vi "zmq_recv_multi.vi"(3 "error in":errorcluster, 5 "socket in":refnum<class "zmq_socket.lvclass">) -> (0 "error out":errorcluster, 1 "parts":string[](array[string]), 2 "socket out":refnum<class "zmq_socket.lvclass">)   [LabVIEW 2019, in "zeromq.lvlib" / "zmq_socket.lvclass"]
doc: "Receive a multi-component message from the socket. The incoming messages are returned as an array of strings, with one string for each message part.\n\nIf <b>no block?</b> is True, the function call will return immediately. Use zmq_check_timeout to see if it was simply a timeout or an error occurred.\n\nOtherwise this call will block until <b>all</b> parts of the message are received, an error is raised, or the socket is closed.\n\nNote there is no penalty using this function to receive single-part messages.\n\nDetailed API documentation: http://api.zeromq.org/3-2:zmq-recv"
uses:
  zmq_socket.lvclass
  zmq_socket.lvclass/zmq_socket.ctl
  <vilib>/Utility/error.llb/Error Cluster From Error Code.vi
  zeromq.lvlib
panel:
  # "ØMQ"
  # "labview"
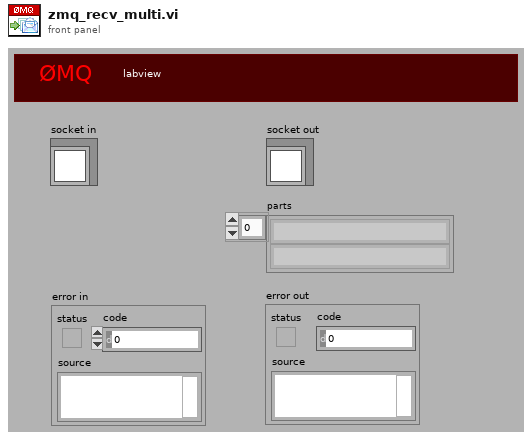
[diagram p1: front panel]
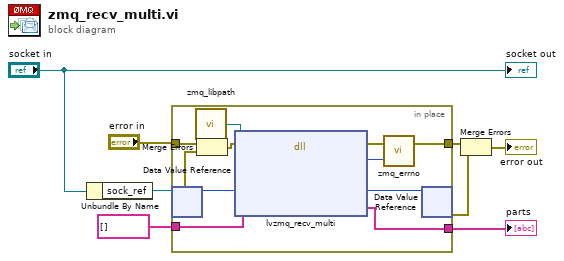
[diagram p0: block diagram]
diagram:
  n1 = Unbundle By Name("socket in") -> ("sock_ref"=w4:refnum<data-value>)
  n2 = in-place {
    in-place-border: "error in" -> [w17]
    in-place-border: [w16] -> w7
    in-place-border: string[] [] ("parts") -> [w15]
    in-place-border: [w12] -> w3
    n3 = in-place-dvr #1(w4) -> (w14:u64, w9:errorcluster)
    n4 = call "zmq_libpath.vi"() -> ("path"=w11:path)
    n5 = Merge Errors(w17, w9) -> (w10:errorcluster)
    n6 = dll-call lib="?" fn="lvzmq_recv_multi" ("zmq_labview.dll:lvzmq_socket")(path in=w11, error in=w10, "sock_obj"=w14, "data"=w15) -> (error out=w19:errorcluster, "return type"=w18:i32, "sock_obj"=w13:u64, "data"=w12:string[])  [unwired: 3 in, 1 out]
    n7 = call "zmq_errno.vi"("retval"=w18, "error in"=w19) -> ("error out"=w16:errorcluster)  [unwired: 1 out]
    n8 = in-place-dvr #1(w13) -> (w1:errorcluster)  [unwired: 1 out]
  }
  "parts" <- w3
  n9 = Merge Errors(w7, w1) -> (→"error out":errorcluster)
  "socket out" <- "socket in"
